vi "Verify with Regex Scrubber.vi"(8 "error in":errorcluster) -> (0 "error out":errorcluster)   [LabVIEW 2020, in "Scrubber.Tests.lvclass"]
uses:
  Scrubber.Tests.lvclass
  Scrubber.Tests.lvclass/Scrubber.Tests.ctl
  <vilib>/addons/_JKI Toolkits/Caraya/classes/Test/Test.lvclass
  4b862e9e-fcb2-487f-ab73-d9f83fbf4d2c.vi
  Source/Approval Tests/Regex Scrubber/Regex Scrubber.lvclass
  Source/Approval Tests/Options/Options.lvclass
  C:/Users/SAS/Desktop/ApprovalTests.LabVIEW/Source/Approval Tests/Scrubber/Scrubber.lvclass
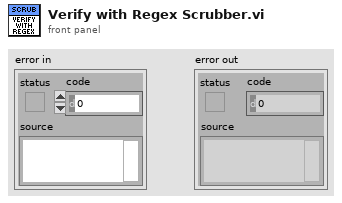
[diagram p1: front panel]
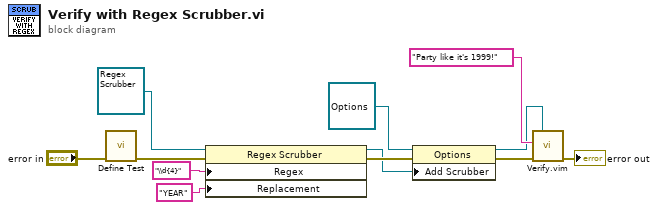
[diagram p0: block diagram]
diagram:
  n1 = call <vilib>:"Define Test.vi"("error in (no error)"="error in") -> ("error out"=w12:errorcluster)  [unwired: 9 in, 1 out]
  n2 = property class="Regex Scrubber"(reference=refnum<class "Regex Scrubber.lvclass"> refnum ("Approval Tests.lvlib:Regex Scrubber.lvclass"), error in=w12, "Regex"="\\d{4}", "Replacement"="YEAR") -> (reference out=w2:refnum<class "Regex Scrubber.lvclass">, error out=w9:errorcluster)
  n3 = property class="Options"(reference=refnum<class "Options.lvclass"> refnum ("Approval Tests.lvlib:Options.lvclass"), error in=w9, "Add Scrubber"=w2) -> (reference out=w1:refnum<class "Options.lvclass">, error out=w8:errorcluster)
  n4 = call "Verify.vim"("Options"=w1, "error in"=w8, "Test Data"="Party like it's 1999!") -> ("error out"=→"error out":errorcluster)  [unwired: 7 in, 1 out]
